vi "GetSVNRevision.vi"(11 "File Path Control":path caption="File Path Control (leave blank to use Constants_Global value of EnFlo SW Folder)") -> (0 "info&status error":string, 1 "LocalModifications":string, 2 "branch":string, 3 "OverallRevision":string, 4 "Brief Output":string, 5 "info&status output":string)   [LabVIEW 2022 SP3]
doc: "This VI uses the system's installed svn (subversion) software to return the revision number of the selected folder. Leaving the selected folder blank will use the global value of \"EnFlo SW Folder\".\nThe \"Overall Revision\" is the highest revision number in the entire hierarchy, recursing upwards as well as downwards- in other words, the revision which was checked out. The \"This Folder\" data is specific to the last changes to the selected folder."
uses:
  <vilib>/Utility/error.llb/Trim Whitespace One-Sided.vi
  Globals/Constants_global.vi
  <vilib>/regexp/Match Regular Expression.xnode
panel:
  out "standard output":string
  out "This Folder's Last Changed Date":string
  out "This Folder Last Committed By":string
  out "This Folder's Last Revision":string
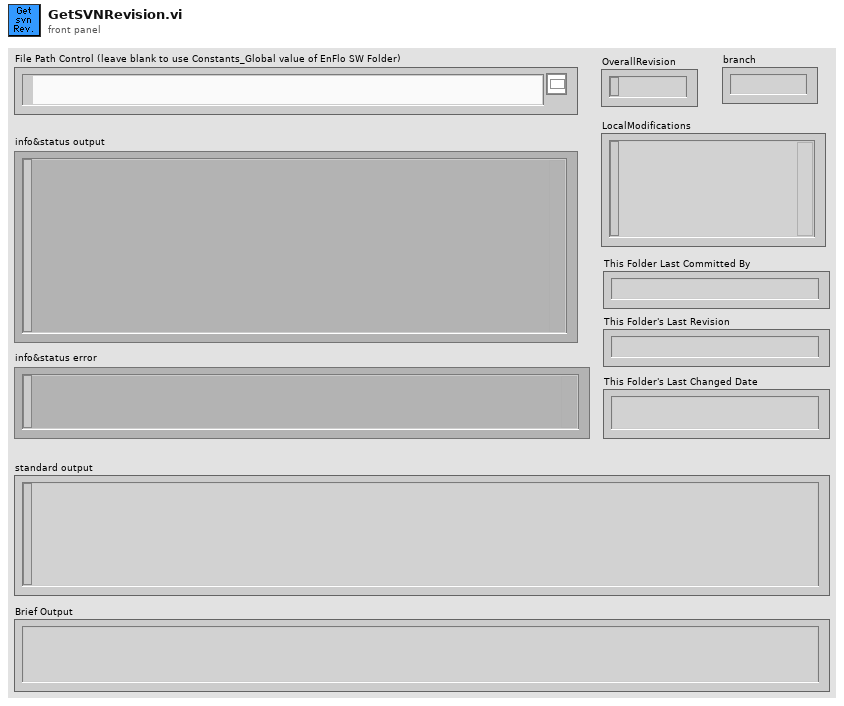
[diagram p1: front panel]
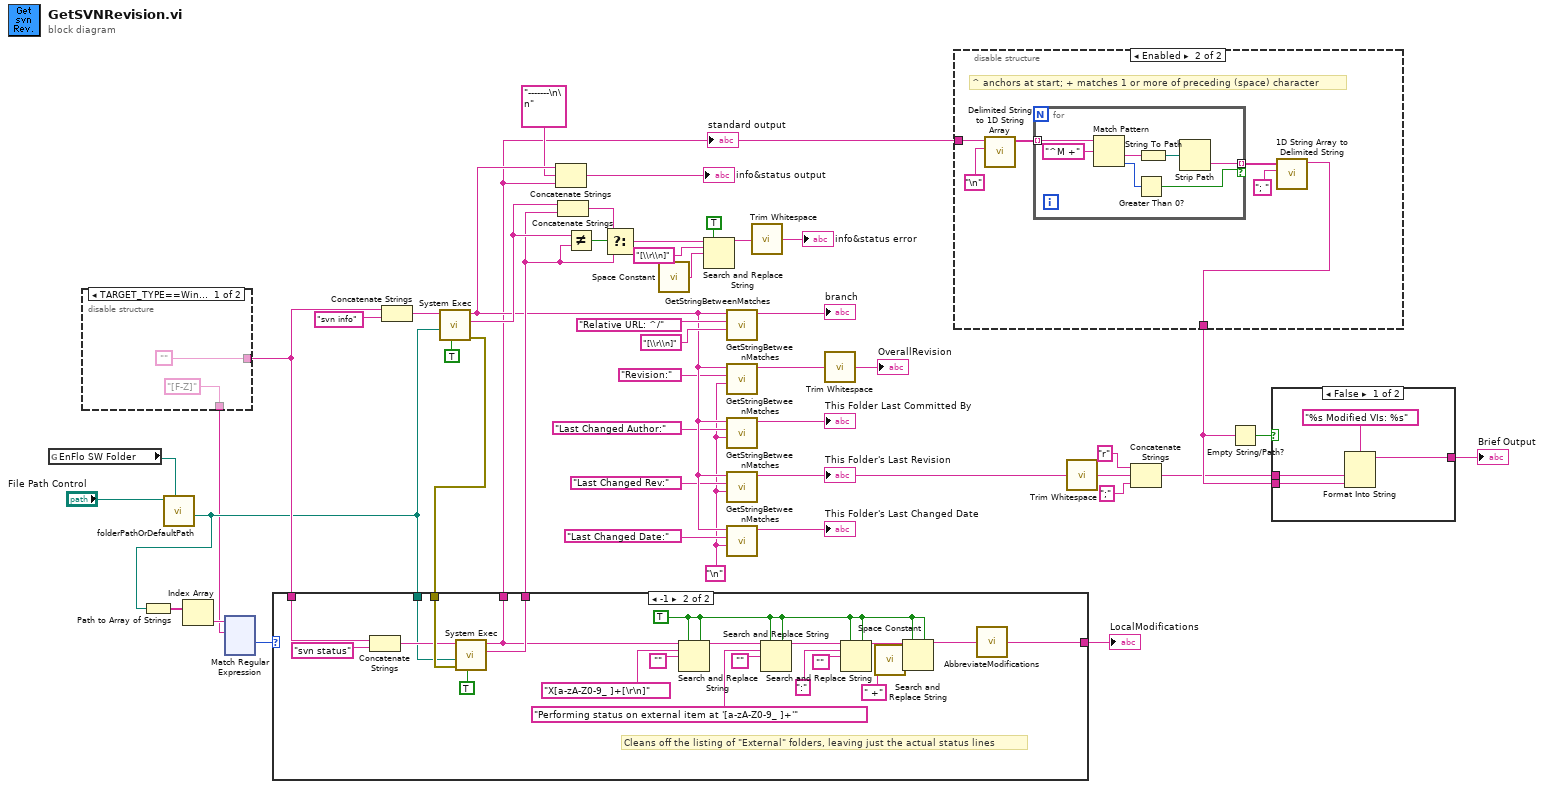
[diagram p0: block diagram]
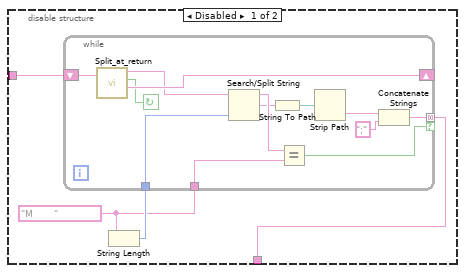
[diagram p2: hidden frame]
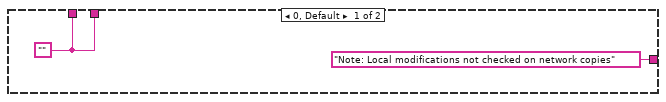
[diagram p4: hidden frame]
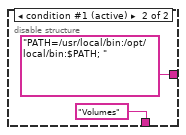
[diagram p5: hidden frame]
diagram:
  w20 = "\n" ("regular expression")
  n1 = global read "Constants_global.vi" "EnFlo SW Folder"() -> (w29:path)
  n2 = disable-structure shown="TARGET_TYPE==Windows, Default" {
    disable-tunnel: ["" ("command line") "PATH=/usr/local/bin:/opt/local/bin:$PATH; " ("command line")] -> w33
    disable-tunnel: ["[F-Z]" ("regular expression") "Volumes" ("regular expression")] -> w10
    frame condition #0 {
    }
    frame condition #1 (active) {
    }
  }
  n3 = call "folderPathOrDefaultPath.vi"("defaultPath"=w29, "File Path Control"="File Path Control") -> ("folder"=w14:path)  [unwired: 8 in, 1 out]
  n4 = Path to Array of Strings(0:w14) -> (2:w13:string[])  [unwired: 1 out]
  n5 = Index Array(array=w13) -> (element=w12:string)  [unwired: 1 in]
  n6 = xnode "Match Regular Expression"("input string"=w12, "regular expression"=w10) -> ("offset past match"=w11:i32)  [unwired: 4 in, 4 out]
  n7 = Concatenate Strings(w33, "svn info" ("command line")) -> (w35:string)
  n8 = call <vilib>:"System Exec.vi"("run minimized? (F)"=TRUE, "working directory"=w14, "command line"=w35) -> ("error out"=w47:errorcluster, "standard error"=w44:string, "standard output"=w25:string)  [unwired: 5 in, 1 out]
  n9 = case shown="-1" w11 {
    tunnel: w47 -> [_ w74]
    tunnel: [w53 w73] -> w41
    tunnel: w33 -> [_ w58]
    tunnel: w14 -> [_ w57]
    tunnel: [w53 w56] -> w4
    tunnel: ["Note: Local modifications not checked on network copies" ("VInames") w54] -> w15
    frame 0, Default {
      w53 = ""
    }
    frame -1 {
      w63 = TRUE ("replace all? (F)")
      # "Cleans off the listing of \"External\" folders, leaving just the actual status lines"
      n10 = Concatenate Strings(w58, "svn status" ("command line")) -> (w60:string)
      n11 = call <vilib>:"System Exec.vi"("run minimized? (F)"=TRUE, "error in (no error)"=w74, "working directory"=w57, "command line"=w60) -> ("standard error"=w73:string, "standard output"=w56:string)  [unwired: 4 in, 2 out]
      n12 = Search and Replace String(replace all?=w63, multiline?=w63, input string=w56, search string="X[a-zA-Z0-9_ ]+[\r\n]", replace string="") -> (result string=w69:string)  [unwired: 3 in, 3 out]
      n13 = Search and Replace String(replace all?=w63, multiline?=w63, input string=w69, search string="Performing status on external item at '[a-zA-Z0-9_ ]+'", replace string="") -> (result string=w67:string)  [unwired: 3 in, 3 out]
      n14 = Search and Replace String(replace all?=w63, multiline?=w63, input string=w67, search string=":", replace string="") -> (result string=w64:string)  [unwired: 3 in, 3 out]
      n15 = call <vilib>:"Space Constant.vi"() -> ("String"=w61:string)
      n16 = Search and Replace String(replace all?=w63, multiline?=w63, input string=w64, search string=" +", replace string=w61) -> (result string=w55:string)  [unwired: 3 in, 3 out]
      n17 = call "AbbreviateModifications.vi"("svnString"=w55) -> ("VInames"=w54:string)  [unwired: 4 in]
    }
  }
  "LocalModifications" <- w15
  "standard output" <- w4
  n18 = Concatenate Strings(w25, "-------\n\n" ("string"), w4) -> (→"info&status output":string)
  n19 = Concatenate Strings(w44, w41) -> (w42:string)
  n20 = Not Equal?(x=w44, y=w41) -> (x != y?=w43:bool)
  n21 = Select(t=w42, s=w43, f=w41) -> (s? t:f=w37:string)
  n22 = call <vilib>:"Space Constant.vi"() -> ("String"=w39:string)
  n23 = Search and Replace String(replace all?=TRUE ("replace all? (F)"), input string=w37, search string="[\\r\\n]", replace string=w39) -> (result string=w36:string)  [unwired: 4 in, 3 out]
  n24 = call "GetStringBetweenMatches.vi"("postTarget"="[\\r\\n]" ("regular expression"), "preTarget"="Relative URL: ^/" ("regular expression"), "stringIn"=w25) -> ("target"=→"branch":string)  [unwired: 7 in, 1 out]
  n25 = call "GetStringBetweenMatches.vi"("postTarget"=w20, "preTarget"="Revision:" ("regular expression"), "stringIn"=w25) -> ("target"=w19:string)  [unwired: 7 in, 1 out]
  n26 = call "GetStringBetweenMatches.vi"("postTarget"=w20, "preTarget"="Last Changed Author:" ("regular expression"), "stringIn"=w25) -> ("target"=→"This Folder Last Committed By":string)  [unwired: 7 in, 1 out]
  n27 = call "GetStringBetweenMatches.vi"("postTarget"=w20, "preTarget"="Last Changed Rev:" ("regular expression"), "stringIn"=w25) -> ("target"=w6:string)  [unwired: 7 in, 1 out]
  "This Folder's Last Revision" <- w6
  n28 = call "GetStringBetweenMatches.vi"("postTarget"=w20, "preTarget"="Last Changed Date:" ("regular expression"), "stringIn"=w25) -> ("target"=→"This Folder's Last Changed Date":string)  [unwired: 7 in, 1 out]
  n29 = call <vilib>:"Trim Whitespace.vi"("string"=w36) -> ("trimmed string"=→"info&status error":string)  [unwired: 1 in]
  n30 = call <vilib>:"Trim Whitespace.vi"("string"=w19) -> ("trimmed string"=→"OverallRevision":string)  [unwired: 1 in]
  n31 = disable-structure shown="Enabled" {
    disable-tunnel: [w77 w93] -> w7
    disable-tunnel: w4 -> [w76 w94]
    frame Disabled {
      w78 = "M       "
      n32 = String Length(string=w78) -> (length=w79:i32)
      n33 = while {
        shift-right: [w91] -> _
        shift-left: w76 -> [w92]
        tunnel: w79 -> [w86]
        tunnel: w78 -> [w89]
        tunnel: [w80] -> w77 mode=concatenating if=w88
        stop <- w90 continue-if-true
        n34 = call "Split_at_return.vi"("String"=w92) -> ("before substring"=w87:string, "Matched?"=w90:bool, "after substring"=w91:string)  [unwired: 1 in, 1 out]
        n35 = Search/Split String(string=w87, offset (0)=w86) -> (substring before match=w85:string, match + rest of string=w84:string)  [unwired: 1 in, 1 out]
        n36 = String To Path(string=w84) -> (path=w83:path)
        n37 = Equal?(x=w85, y=w89) -> (x = y?=w88:bool)
        n38 = Strip Path(path=w83) -> (name=w82:string)  [unwired: 1 out]
        n39 = Concatenate Strings(w82, ";" ("string")) -> (w80:string)
      }
    }
    frame Enabled {
      # "^ anchors at start; + matches 1 or more of preceding (space) character"
      n40 = call <vilib>:"Delimited String to 1D String Array.vi"("delimiter"="\n", "delimited string"=w94) -> ("string array"=w97:string[])  [unwired: 9 in]
      n41 = for {
        tunnel: w97 -> [w105] mode=indexing
        tunnel: [w100] -> w98 mode=indexing if=w99
        n42 = Match Pattern(string=w105, regular expression="^M +") -> (after substring=w102:string, offset past match=w103:i32)  [unwired: 1 in, 2 out]
        n43 = Greater Than 0?(x=w103) -> (x > 0?=w99:bool)
        n44 = String To Path(string=w102) -> (path=w101:path)
        n45 = Strip Path(path=w101) -> (name=w100:string)  [unwired: 1 out]
      }
      n46 = call <vilib>:"1D String Array to Delimited String.vi"("delimiter"="; ", "string array"=w98) -> ("delimited string"=w93:string)  [unwired: 9 in]
    }
  }
  n47 = call <vilib>:"Trim Whitespace.vi"("string"=w6) -> ("trimmed string"=w5:string)  [unwired: 1 in]
  n48 = Concatenate Strings("r" ("string"), w5, ";" ("string")) -> (w3:string)
  n49 = Empty String/Path?(string/path=w7) -> (empty?=w9:bool)
  n50 = case shown="False" w9 {
    tunnel: [w106 w110] -> w8
    tunnel: w3 -> [w108 w110]
    tunnel: w7 -> [w107 _]
    frame False {
      n51 = Format Into String(format string="%s Modified VIs: %s", w108, w107) -> (resulting string=w106:string)  [unwired: 2 in, 1 out]
    }
    frame True {
    }
  }
  "Brief Output" <- w8
